vi "Source Directory.vi"() -> (0 "Source Directory":path)   [LabVIEW 2017]
doc: "Gets the \"src\" directory relative to the project root."
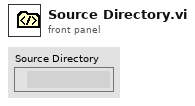
[diagram p1: front panel]
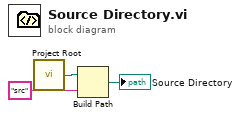
[diagram p0: block diagram]
diagram:
  n1 = call "Project Root.vi"() -> ("Project Root"=w1:path)
  n2 = Build Path(base path=w1, name or relative path="src") -> (appended path=→"Source Directory":path)
